vi "Main.vi"(6 "Folder names":string[](array[string])=["StaARx#[PLC]StaATesterRxSignals", "StaATx#[PLC]StaATesterTxSignals"], 8 "error in":errorcluster, 9 "Sequence Context":refnum<k7>, 10 "OPC UA refnum":T1, 11 "OPC UA In":refnum<class "OPC UA.lvclass">) -> (0 "error out":errorcluster, 3 "OPC UA Out":refnum<class "OPC UA.lvclass">)   [LabVIEW 2019, in "OPC UA.lvlib" / "OPC UA.lvclass"]
uses:
  OPC UA.lvclass
  Tester Rx Dataset.ctl
  Tester Tx Dataset.ctl
  OPC UA.lvclass/OPC UA.ctl
  <vilib>/OPCUA/NI OPC UA Client.lvlib
  <vilib>/OPCUA/controls/OPC UA Client Refnum.ctl
panel:
  in  "Tx to PLC":T2
  out "Rx from PLC":T3={"Start"=FALSE, "NestStatus"=FALSE, "PalletID"=0, "BarcodeData"="P:10-000001R:04S:QMC2200001", "StepEcho"=0, "Cylinder_1"=FALSE, "Cylinder_2"=FALSE, "Cylinder_3"=FALSE, "Cylinder_4"=FALSE, "Cylinder_5"=FALSE, "ResultsAck"=FALSE, "Reset"=FALSE, "Stop"=FALSE, "FaultCode"=0}
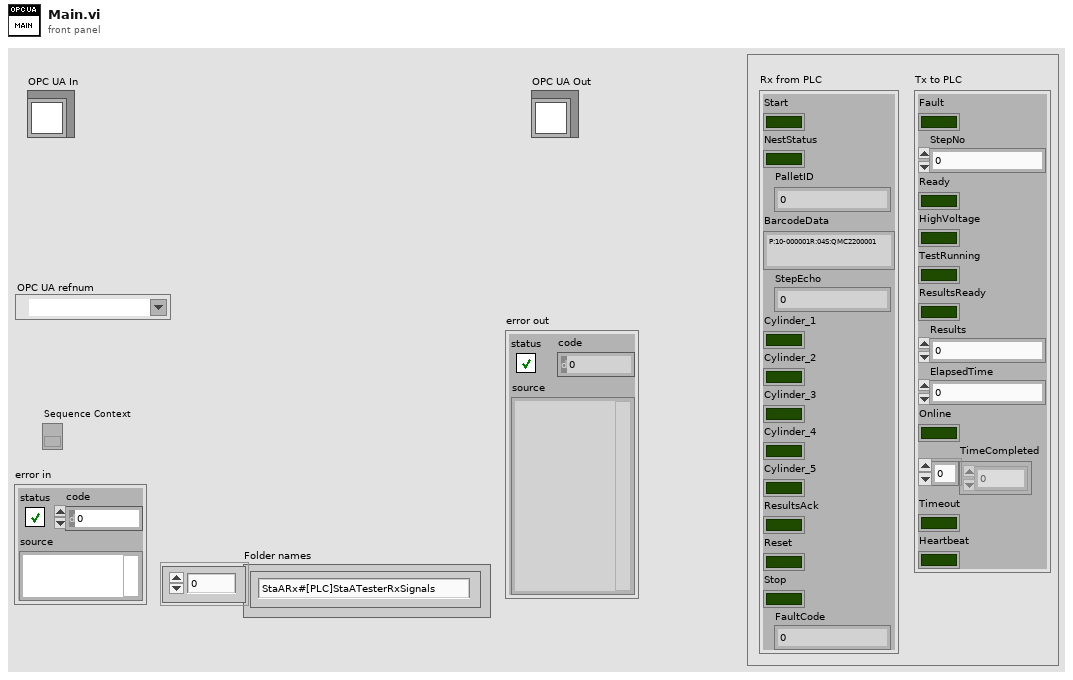
[diagram p1: front panel]
types:
  T1 = typedef "OPC UA Client Refnum.ctl" = refnum<k21>
  T2 = typedef "OPC UA.lvlib/OPC UA.lvclass/Tester Tx Dataset.ctl" = cluster{"Fault":bool, "StepNo":u32, "Ready":bool, "HighVoltage":bool, "TestRunning":bool, "ResultsReady":bool, "Results":u32, "ElapsedTime":u32, "Online":bool, "TimeCompleted":i32[], "Timeout":bool, "Heartbeat":bool}
  T3 = typedef "OPC UA.lvlib/OPC UA.lvclass/Tester Rx Dataset.ctl" = cluster{"Start":bool, "NestStatus":bool, "PalletID":u32, "BarcodeData":string, "StepEcho":u32, "Cylinder_1":bool, "Cylinder_2":bool, "Cylinder_3":bool, "Cylinder_4":bool, "Cylinder_5":bool, "ResultsAck":bool, "Reset":bool, "Stop":bool, "FaultCode":u32}
  T4 = typedef "Subscription ID.ctl" = u32
  T5 = typedef "TestStand - Status Monitor.ctl" = cluster{"Sequence Context":refnum<k7>, "Execution":refnum<k7>, "Termination Monitor":refnum<k7>}
  T6 = cluster{"Event Registration Refnum":refnum<event-registration>, "Event Registration Refnum":refnum<event-registration>}
  T7 = typedef "Subscription Data Change.ctl" = cluster{"node ID":T8, " value":variant, "timestamp":timestamp, "data type":T9, "status code":T10}
  T8 = typedef "NodeId.ctl" = string
  T9 = typedef "Data Type.ctl" = u16
  T10 = typedef "OPC UA StatusCode.ctl" = u32
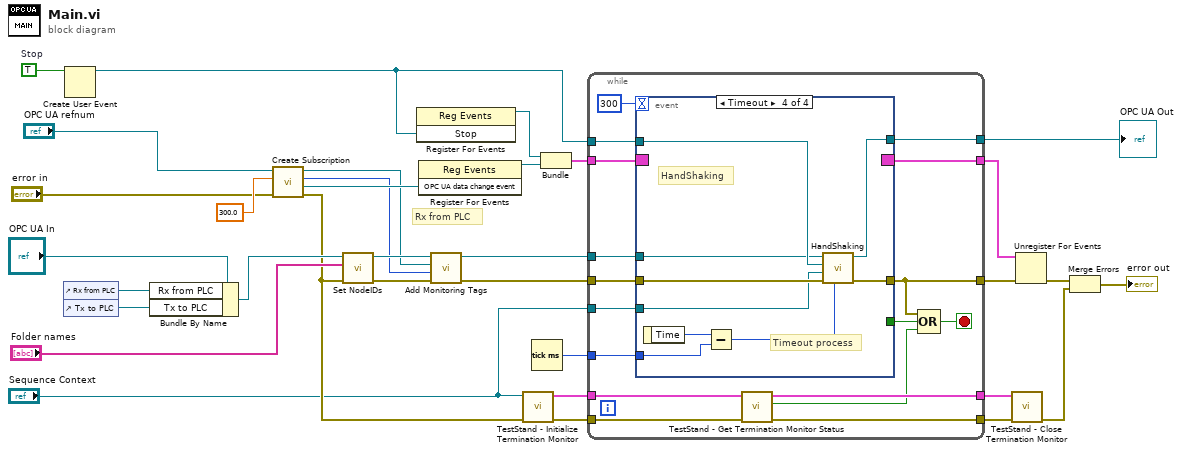
[diagram p0: block diagram]
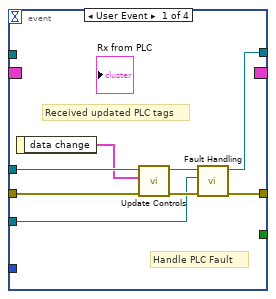
[diagram p2: hidden frame]
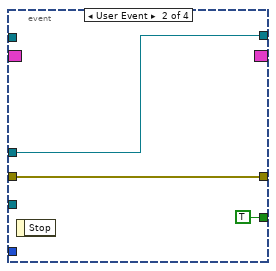
[diagram p3: hidden frame]
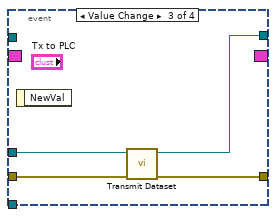
[diagram p4: hidden frame]
diagram:
  w6 = TRUE  # Stop
  # "Rx from PLC"
  n1 = control-ref of="Rx from PLC"() -> (w13:refnum<vi>)
  n2 = control-ref of="Tx to PLC"() -> (w11:refnum<vi>)
  n3 = Create User Event(user event datatype=w6) -> (user event=w5:refnum<user-event>)  [unwired: 1 in, 1 out]
  n4 = Bundle By Name(cluster="OPC UA In", "Rx from PLC"=w13, "Tx to PLC"=w11) -> (w12:refnum<class "OPC UA.lvclass">)
  n5 = call <vilib>:"Create Subscription.vi"("error in (no error)"="error in", "publishing interval (1000 ms)"=300.0, "OPC UA client refnum in"="OPC UA refnum") -> ("error out"=w7:errorcluster, "OPC UA data change event"=w18:refnum<user-event>, "subscription ID out"=w17:T4, "OPC UA client refnum out"=w16:T1)  [unwired: 4 in, 1 out]
  n6 = call "Set NodeIDs.vi"("error in (no error)"=w7, "PLC Folder Names"="Folder names", "OPC UA in"=w12) -> ("error out"=w32:errorcluster, "OPC UA out"=w31:refnum<class "OPC UA.lvclass">)  [unwired: 7 in]
  n7 = register-events(w5) -> (reference out=w8:refnum<event-registration>)  [unwired: 2 in, 1 out]
  n8 = register-events(w18) -> (reference out=w10:refnum<event-registration>)  [unwired: 2 in, 1 out]
  n9 = call "Add Monitoring Tags.vi"("error in (no error)"=w32, "subscription ID"=w17, "OPC UA client refnum"=w16, "OPC UA in"=w31) -> ("error out"=w15:errorcluster, "OPC UAout"=w20:refnum<class "OPC UA.lvclass">)  [unwired: 6 in]
  n10 = call <vilib>:"TestStand - Initialize Termination Monitor.vi"("error in (no error)"=w7, "Sequence Context In"="Sequence Context") -> ("error out"=w30:errorcluster, "Status Monitor Out"=w29:T5)  [unwired: 8 in]
  n11 = Tick Count (ms)() -> (millisecond timer value=w23:u32)
  n12 = Bundle("Event Registration Refnum"=w8, "Event Registration Refnum"=w10) -> (w9:T6)  [unwired: 1 in]
  n13 = while {
    tunnel: w9 -> [w36]
    tunnel: w20 -> [w50]
    tunnel: w15 -> [w49]
    tunnel: [w38] -> w26
    tunnel: [w47] -> w25
    tunnel: w30 -> [w46]
    tunnel: w29 -> [w45]
    tunnel: [w43] -> w28
    tunnel: [w42] -> w27
    tunnel: [w41] -> w14
    tunnel: w23 -> [w40]
    tunnel: w5 -> [w35]
    tunnel: "Sequence Context" -> [w34]
    stop <- w44 stop-if-true
    n14 = event shown="[3] Timeout" {
      selector: w36 -> [_ _ _ _]
      dyn-events: [_ _ _ _] -> w47
      timeout: 300 -> [_ _ _ _]
      tunnel: w50 -> [w58 w61 w63 w67]
      tunnel: w49 -> [w57 w60 w64 w72]
      tunnel: [w55 w60 w65 w74] -> w38
      tunnel: [w54 w61 w62 w73] -> w41
      tunnel: w40 -> [_ _ _ w70]
      tunnel: [_ TRUE ("Stop") _ _] -> w37
      tunnel: w35 -> [_ _ _ w68]
      tunnel: w34 -> [w51 _ _ w66]
      event User Event {
        # "Handle PLC Fault"
        # "Received updated PLC tags"
        n15 = event-data() -> ("data change"=w52:T7[])  [unwired: 1 in]
        n16 = call "Update Controls.vi"("error in (no error)"=w57, "data change"=w52, "OPC UA in"=w58) -> ("error out"=w56:errorcluster, "OPC UA out"=w53:refnum<class "OPC UA.lvclass">)  [unwired: 7 in]
        n17 = call "Fault Handling.vi"("error in (no error)"=w56, "Sequence Context"=w51, "OPC UA in"=w53) -> ("error out"=w55:errorcluster, "OPC UA out"=w54:refnum<class "OPC UA.lvclass">)  [unwired: 7 in]
      }
      event User Event {
        n18 = event-data() -> ()  [unwired: 1 in, 1 out]
      }
      event Value Change {
        n19 = event-data() -> ()  [unwired: 1 in, 1 out]
        n20 = call "Transmit Dataset.vi"("error in (no error)"=w64, "OPC UA in"=w63) -> ("error out"=w65:errorcluster, "OPC UA out"=w62:refnum<class "OPC UA.lvclass">)  [unwired: 8 in]
      }
      event Timeout {
        # "HandShaking"
        # "Timeout process"
        n21 = event-data() -> ("Time"=w71:u32)  [unwired: 1 in]
        n22 = Subtract(x=w71, y=w70) -> (x-y=w69:u32)
        n23 = call-dynamic "HandShaking.vi"("Elapsed Time"=w69, "error in (no error)"=w72, "Sequence Context"=w66, "Stop"=w68, "OPC UA in"=w67) -> ("error out"=w74:errorcluster, "OPC UA out"=w73:refnum<class "OPC UA.lvclass">)  [unwired: 5 in]
      }
    }
    n24 = call <vilib>:"TestStand - Get Termination Monitor Status.vi"("error in (no error)"=w46, "Status Monitor In"=w45) -> ("error out"=w43:errorcluster, "Terminating or Aborting"=w39:bool, "Status Monitor Out"=w42:T5)  [unwired: 7 in]
    n25 = Compound Arithmetic op=OR(w38, w37, w39) -> (w44:bool)
  }
  "OPC UA Out" <- w14
  n26 = call <vilib>:"TestStand - Close Termination Monitor.vi"("error in (no error)"=w28, "Status Monitor In"=w27) -> ("error out"=w21:errorcluster)  [unwired: 9 in]
  n27 = Unregister For Events(event registration refnum=w25, error in=w26) -> (error out=w22:errorcluster)
  n28 = Merge Errors(w22, w21) -> (→"error out":errorcluster)
